vi "Concatenate DUT results.vi"(10 "Acquire Testing":T2, 11 "DUT":T1) -> (3 "DUT with added Results":T1)   [LabVIEW 2023]
uses:
  Queue/DUTinfo.ctl
  Queue/DUTResult.ctl
  Queue/Queue Priority.ctl
  Queue/Queues.lvlib
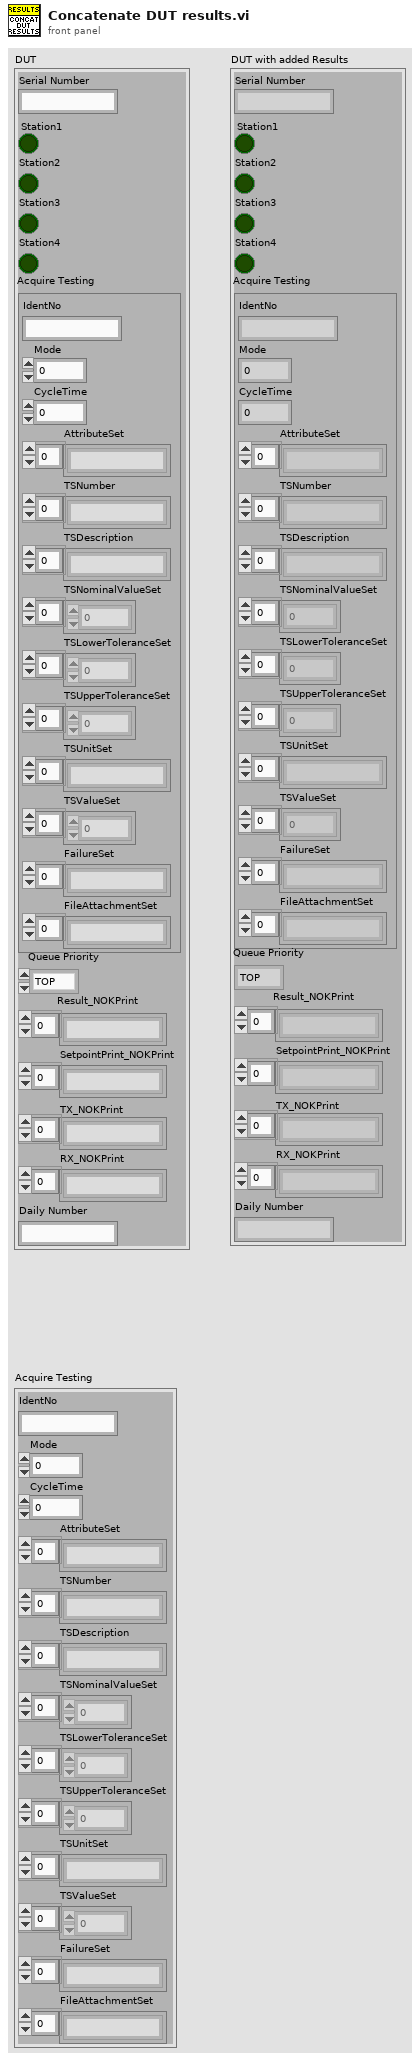
[diagram p1: front panel]
types:
  T1 = typedef "Queues.lvlib/DUTinfo.ctl" = cluster{"Serial Number":string, "Station1":bool, "Station2":bool, "Station3":bool, "Station4":bool, "Acquire Testing":T2, "Queue Priority":T3, "Result_NOKPrint":string[], "SetpointPrint_NOKPrint":string[], "TX_NOKPrint":string[], "RX_NOKPrint":string[], "Daily Number":string}
  T2 = typedef "Queues.lvlib/DUTResult.ctl" = cluster{"IdentNo":string, "Mode":dbl, "CycleTime":dbl, "AttributeSet":string[], "TSNumber":string[], "TSDescription":string[], "TSNominalValueSet":dbl[], "TSLowerToleranceSet":dbl[], "TSUpperToleranceSet":dbl[], "TSUnitSet":string[], "TSValueSet":dbl[], "FailureSet":string[], "FileAttachmentSet":string[]}
  T3 = typedef "Queues.lvlib/Queue Priority.ctl" = enum16{"TOP", "BOTTOM"}
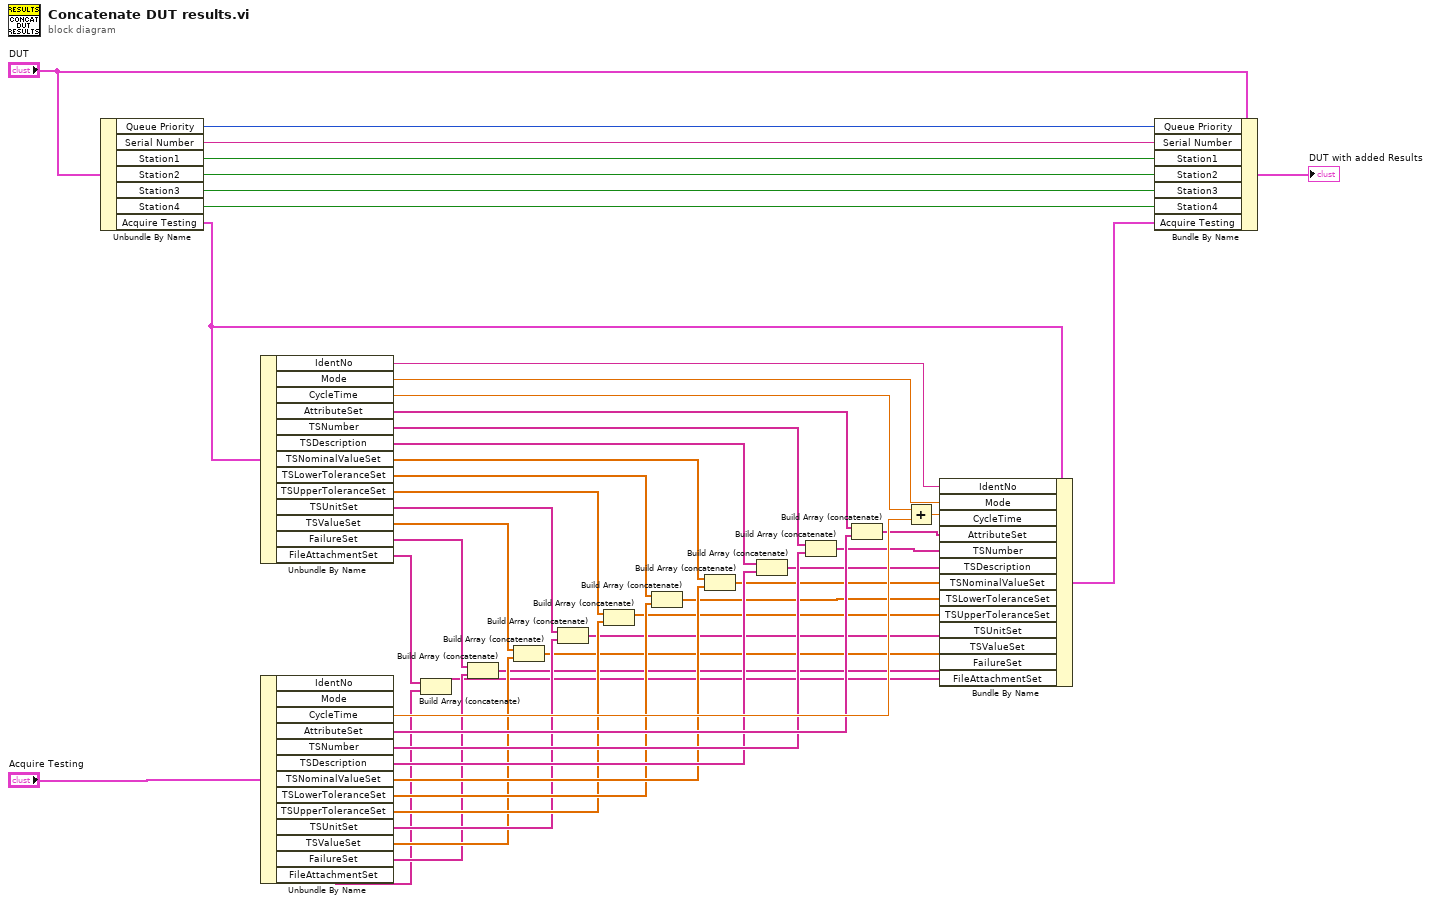
[diagram p0: block diagram]
diagram:
  n1 = Unbundle By Name("DUT") -> ("Queue Priority"=w9:T3, "Serial Number"=w8:string, "Station1"=w7:bool, "Station2"=w6:bool, "Station3"=w5:bool, "Station4"=w4:bool, "Acquire Testing"=w2:T2)
  n2 = Unbundle By Name(w2) -> ("IdentNo"=w44:string, "Mode"=w43:dbl, "CycleTime"=w41:dbl, "AttributeSet"=w39:string[], "TSNumber"=w36:string[], "TSDescription"=w33:string[], "TSNominalValueSet"=w30:dbl[], "TSLowerToleranceSet"=w27:dbl[], "TSUpperToleranceSet"=w24:dbl[], "TSUnitSet"=w21:string[], "TSValueSet"=w18:dbl[], "FailureSet"=w15:string[], "FileAttachmentSet"=w12:string[])
  n3 = Unbundle By Name("Acquire Testing") -> ("CycleTime"=w40:dbl, "AttributeSet"=w38:string[], "TSNumber"=w35:string[], "TSDescription"=w32:string[], "TSNominalValueSet"=w29:dbl[], "TSLowerToleranceSet"=w26:dbl[], "TSUpperToleranceSet"=w23:dbl[], "TSUnitSet"=w20:string[], "TSValueSet"=w17:dbl[], "FailureSet"=w14:string[], "FileAttachmentSet"=w11:string[])  [unwired: 2 out]
  n4 = Build Array (concatenate)(w12, w11) -> (w10:string[])
  n5 = Build Array (concatenate)(w15, w14) -> (w13:string[])
  n6 = Build Array (concatenate)(w18, w17) -> (w16:dbl[])
  n7 = Build Array (concatenate)(w21, w20) -> (w19:string[])
  n8 = Build Array (concatenate)(w24, w23) -> (w22:dbl[])
  n9 = Build Array (concatenate)(w27, w26) -> (w25:dbl[])
  n10 = Build Array (concatenate)(w30, w29) -> (w28:dbl[])
  n11 = Build Array (concatenate)(w33, w32) -> (w31:string[])
  n12 = Build Array (concatenate)(w36, w35) -> (w34:string[])
  n13 = Build Array (concatenate)(w39, w38) -> (w37:string[])
  n14 = Add(x=w41, y=w40) -> (x+y=w42:dbl)
  n15 = Bundle By Name(cluster=w2, "IdentNo"=w44, "Mode"=w43, "CycleTime"=w42, "AttributeSet"=w37, "TSNumber"=w34, "TSDescription"=w31, "TSNominalValueSet"=w28, "TSLowerToleranceSet"=w25, "TSUpperToleranceSet"=w22, "TSUnitSet"=w19, "TSValueSet"=w16, "FailureSet"=w13, "FileAttachmentSet"=w10) -> (w1:T2)
  n16 = Bundle By Name(cluster="DUT", "Queue Priority"=w9, "Serial Number"=w8, "Station1"=w7, "Station2"=w6, "Station3"=w5, "Station4"=w4, "Acquire Testing"=w1) -> (→"DUT with added Results":T1)
